vi "Suite from Library.vi"(8 "error in (no error)":errorcluster, 10 "Library Path":path, 11 "LUnit Test Suite In":refnum<class "LUnit Test Suite.lvclass">) -> (0 "error out":errorcluster, 3 "LUnit Test Suite Out":refnum<class "LUnit Test Suite.lvclass">)   [LabVIEW 2020, in "Test Suite Factory.lvclass"]
uses:
  LUnit Test Suite/LUnit Test Suite.lvclass
  C:/git/astemes-lunit/source/Core/Runnable/Runnable.lvclass
  LUnit Test Case/LUnit Test Case.lvclass
  LUnit Test Suite/LUnit Test Suite.lvclass/LUnit Test Suite.ctl
  Test Suite Factory.lvclass
  Test Suite Factory.lvclass/Test Suite Factory.ctl
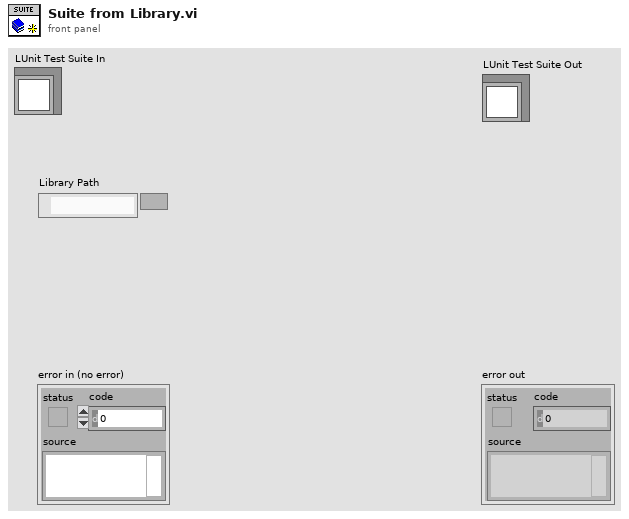
[diagram p1: front panel]
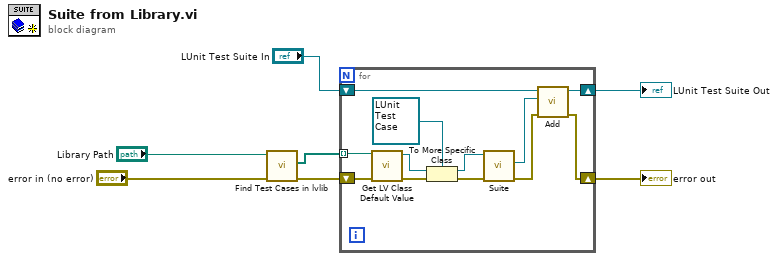
[diagram p0: block diagram]
diagram:
  n1 = call "Find Test Cases in lvlib.vi"("error in (no error)"="error in (no error)", "Project Path"="Library Path") -> ("error out"=w5:errorcluster, "Test Class paths"=w6:path[])  [unwired: 8 in]
  n2 = for {
    tunnel: w6 -> [w13] mode=indexing
    shift-right: [w17] -> w1
    shift-left: "LUnit Test Suite In" -> [w18]
    shift-right: [w12] -> w3
    shift-left: w5 -> [w19]
    n3 = call <vilib>:"Get LV Class Default Value.vi"("error in (no error)"=w19, "class path"=w13) -> ("error out"=w16:errorcluster, "object"=w15:refnum<class>)  [unwired: 8 in]
    n4 = To More Specific Class(target class=refnum<class "LUnit Test Case.lvclass"> refnum ("LUnit Test Case V2.lvclass"), reference=w15, error in=w16) -> (specific class reference=w9:refnum<class "LUnit Test Case.lvclass">, error out=w11:errorcluster)
    n5 = call-dynamic "Suite.vi"("error in (no error)"=w11, "LUnit Test Case in"=w9) -> ("error out"=w10:errorcluster, "LUnit Test Suite Out"=w8:refnum<class "LUnit Test Suite.lvclass">)  [unwired: 7 in, 1 out]
    n6 = call "Add.vi"("error in (no error)"=w10, "Runnable"=w8, "LUnit Test Suite In"=w18) -> ("error out"=w12:errorcluster, "LUnit Test Suite Out"=w17:refnum<class "LUnit Test Suite.lvclass">)  [unwired: 7 in]
  }
  "error out" <- w3
  "LUnit Test Suite Out" <- w1
